vi "LiftMain.vi"(8 "error in (no error)":errorcluster, 9 "Reverse":bool, 10 "Forward":bool, 11 "Control Mode":enum16{"Open", "Control"}(ring)) -> (0 "error out":errorcluster)   [LabVIEW 2016]
uses:
  <vilib>/Rock Robotics/SystemInterfaces/DIO/FPGA_DIORelayChannel.ctl
  <vilib>/Rock Robotics/WPI/Relay/WPI_RelayDirection.ctl
  <vilib>/Rock Robotics/SystemInterfaces/DIO/FPGA_DIOChannel.ctl
  <vilib>/Rock Robotics/WPI/Relay/WPI_RelayValue.ctl
  <vilib>/Rock Robotics/WPI/Switch/WPI_SwitchOpenLimit.vi
  <vilib>/Rock Robotics/Network Tables/NT Read Number.vi
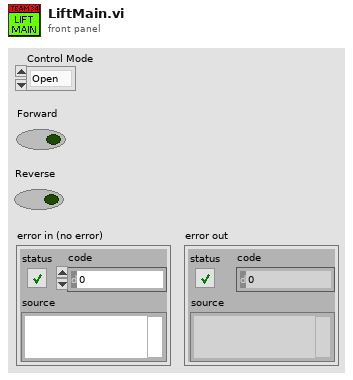
[diagram p1: front panel]
types:
  T1 = typedef "FPGA_DIOChannel.ctl" = enum8{"DIO 0", "DIO 1", "DIO 2", "DIO 3", "DIO 4", "DIO 5", "DIO 6", "DIO 7", "DIO 8", "DIO 9", "DIO MXP 0", "DIO MXP 1", "DIO MXP 2", "DIO MXP 3", "DIO MXP 4", "DIO MXP 5", "DIO MXP 6", "DIO MXP 7", "DIO MXP 8", "DIO MXP 9", "DIO MXP 10", "DIO MXP 11", "DIO MXP 12", "DIO MXP 13", "DIO MXP 14", "DIO MXP 15", "SPI Port CS1", "SPI Port CS2", "SPI Port CS3", "SPI Port MISO", "SPI Port MOSI", "Invalid"}
  T2 = typedef "WPI_RelayDirection.ctl" = enum16{"Both directions", "Forward only", "Reverse only"}
  T3 = typedef "FPGA_DIORelayChannel.ctl" = enum8{"Relay 0", "Relay 1", "Relay 2", "Relay 3", "Invalid"}
  T4 = typedef "WPI_RelayValue.ctl" = enum16{"Off", "On", "Forward", "Reverse"}
  T5 = typedef "WPI_SwitchDevRef.ctl" = cluster{"DevStatus":errorcluster, "DIO Channel":T1, "CntIndex":T6, "Normally Closed":bool}
  T6 = typedef "FPGA_CounterCtrSystemIndex.ctl" = enum8{"Ctr 0", "Ctr 1", "Ctr 2", "Ctr 3", "Ctr 4", "Ctr 5", "Ctr 6", "Ctr 7", "Invalid"}
  T7 = typedef "WPI_RelayDevRef.ctl" = cluster{"DevStatus":errorcluster, "Relay Channel":T3, "Relay Direction":T2}
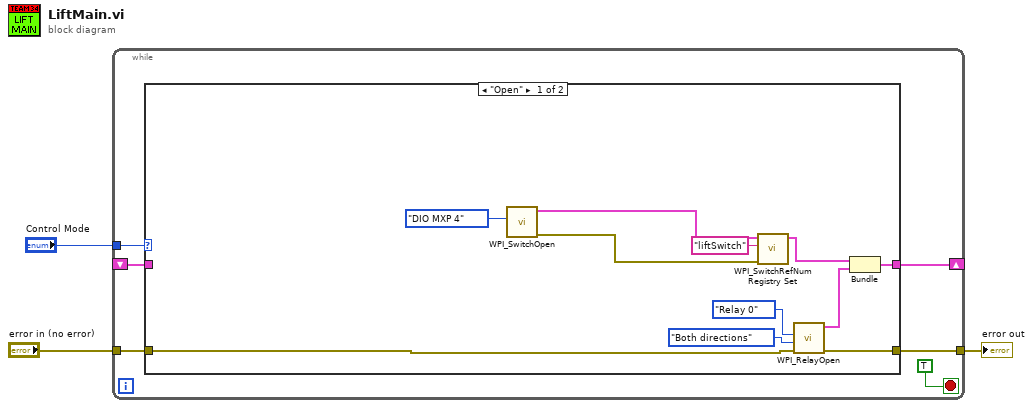
[diagram p0: block diagram]
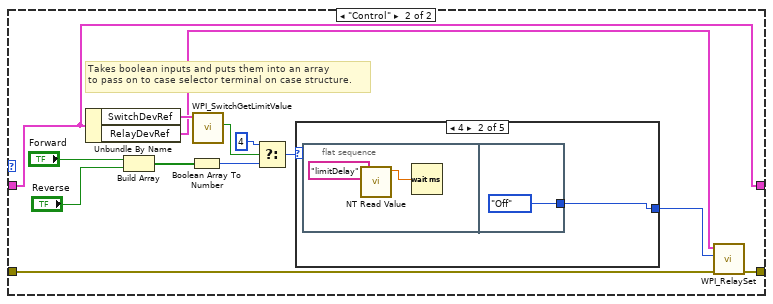
[diagram p2: hidden frame]
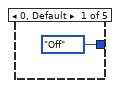
[diagram p3: hidden frame]
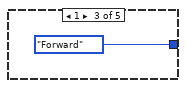
[diagram p4: hidden frame]
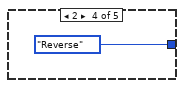
[diagram p5: hidden frame]
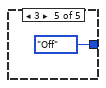
[diagram p6: hidden frame]
diagram:
  n1 = while {
    tunnel: "Control Mode" -> [w8]
    tunnel: "error in (no error)" -> [w7]
    tunnel: [w6] -> w1
    shift-right: [w5] -> _
    shift-left: _ -> [w4]
    stop <- TRUE stop-if-true
    n2 = case shown="\"Open\"" w8 {
      tunnel: w7 -> [w20 w29]
      tunnel: [w19 w30] -> w6
      tunnel: [w14 w25] -> w5
      tunnel: w4 -> [_ w25]
      frame "Open" {
        n3 = call-poly <vilib>:"WPI_SwitchOpen.vi"("DIO Channel"=FPGA_DIOChannel."DIO MXP 4") -> ("error out"=w11:errorcluster, "SwitchDevRef"=w13:T5)  [unwired: 9 in]
        n4 = call <vilib>:"WPI_SwitchRefNum Registry Set.vi"("error in (no error)"=w11, "refnum name"="liftSwitch", "SwitchDevRef"=w13) -> ("SwitchDevRef"=w10:T5)  [unwired: 7 in, 1 out]
        n5 = call <vilib>:"WPI_RelayOpen.vi"("error in (no error)"=w20, "Relay Direction"=WPI_RelayDirection."Both directions", "Relay Channel"=FPGA_DIORelayChannel."Relay 0") -> ("error out"=w19:errorcluster, "RelayDevRef"=w15:T7)  [unwired: 7 in]
        n6 = Bundle("SwitchDevRef"=w10, "RelayDevRef"=w15) -> (w14:cluster{"SwitchDevRef":T5, "RelayDevRef":T7})  [unwired: 1 in]
      }
      frame "Control" {
        # "Takes boolean inputs and puts them into an array\nto pass on to case selector terminal on case structure."
        n7 = Unbundle By Name(w25) -> ("SwitchDevRef"=w23:T5, "RelayDevRef"=w21:T7)
        n8 = Build Array("Forward", "Reverse") -> (w31:bool[])
        n9 = Boolean Array To Number(Boolean array=w31) -> (number=w26:u32)
        n10 = call <vilib>:"WPI_SwitchGetLimitValue.vi"("SwitchDevRef"=w23) -> ("Switch Pressed"=w24:bool)  [unwired: 8 in, 2 out]
        n11 = Select(t=u32 4, s=w24, f=w26) -> (s? t:f=w27:u32)
        n12 = case shown="4" w27 {
          tunnel: [WPI_RelayValue."Off" ("RelayValue") w35 WPI_RelayValue."Forward" ("RelayValue") WPI_RelayValue."Reverse" ("RelayValue") WPI_RelayValue."Off" ("RelayValue")] -> w28
          frame 0, Default {
          }
          frame 4 {
            n13 = flat-sequence {
              tunnel: [WPI_RelayValue."Off" ("RelayValue")] -> w35
              frame #0 {
                n14 = call-poly <vilib>:"NT Read Value.vi"("Name"="limitDelay") -> ("Numeric"=w37:dbl)  [unwired: 9 in, 1 out]
                n15 = Wait (ms)(milliseconds to wait=w37) -> ()  [unwired: 1 out]
              }
              frame #1 {
              }
            }
          }
          frame 1 {
          }
          frame 2 {
          }
          frame 3 {
          }
        }
        n16 = call <vilib>:"WPI_RelaySet.vi"("error in (no error)"=w29, "RelayValue"=w28, "RelayDevRef"=w21) -> ("error out"=w30:errorcluster)  [unwired: 7 in, 1 out]
      }
    }
  }
  "error out" <- w1
